vi "Process Menu Selection.vi"(8 "error in (no error)":errorcluster, 10 "Argument":string, 11 "Menu Ref":refnum<k9>) -> (0 "error out":errorcluster, 3 "State(s) to Enqueue":string)   [LabVIEW 2020, in "VI Properties Editor.lvlib"]
doc: "Processes a menu selection that occurred within the main window."
uses:
  VI Properties Editor.lvlib
  <vilib>/Utility/error.llb/Error Cluster From Error Code.vi
  <vilib>/ErrorRing/Error Ring.xnode
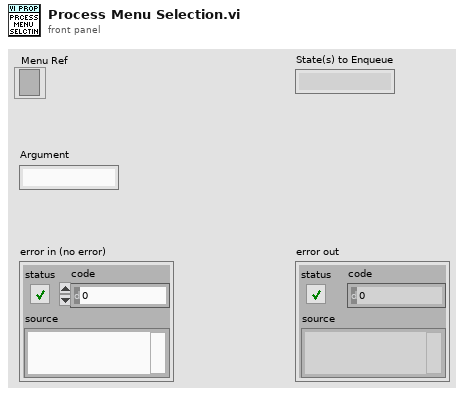
[diagram p1: front panel]
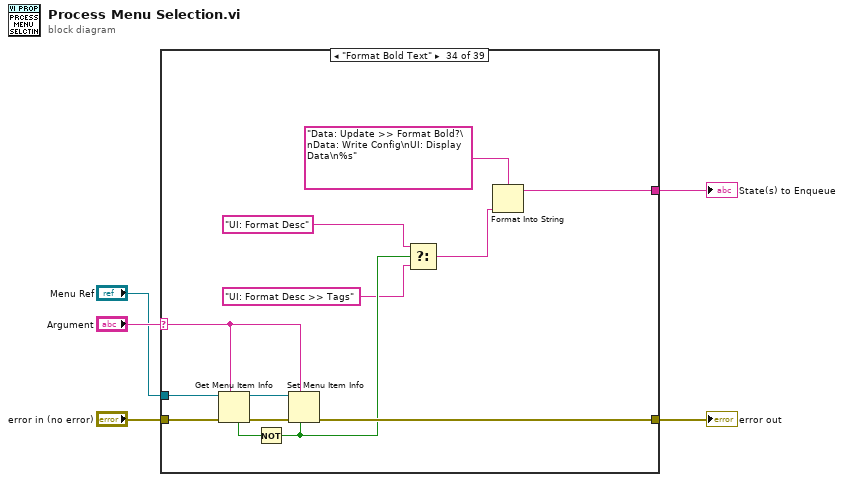
[diagram p0: block diagram]
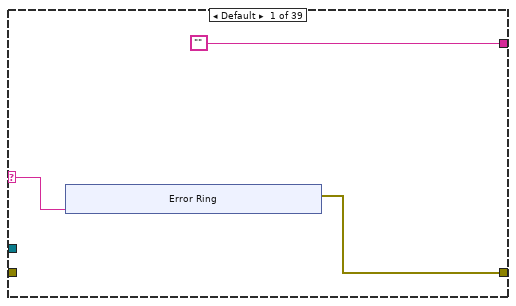
[diagram p2: hidden frame]
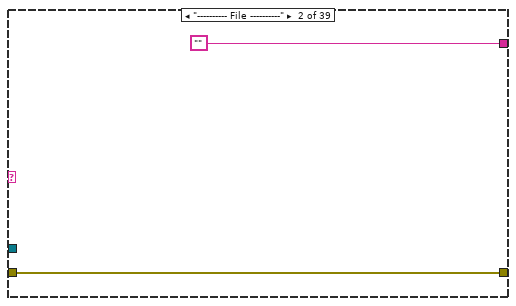
[diagram p3: hidden frame]
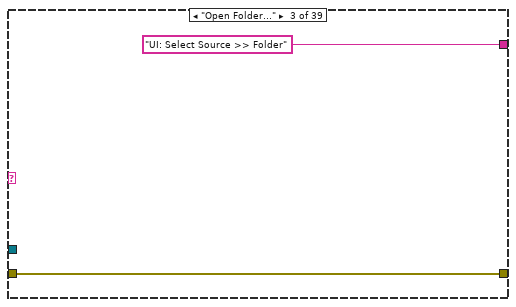
[diagram p4: hidden frame]
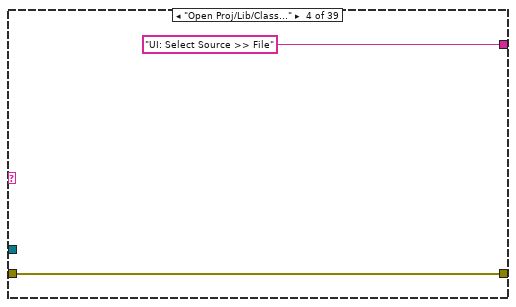
[diagram p5: hidden frame]
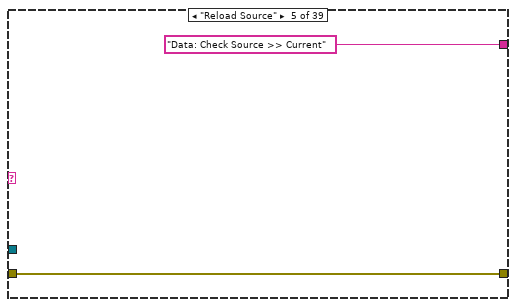
[diagram p6: hidden frame]
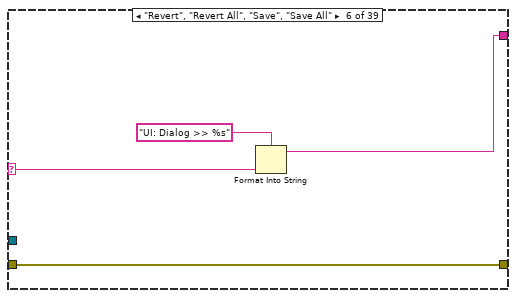
[diagram p7: hidden frame]
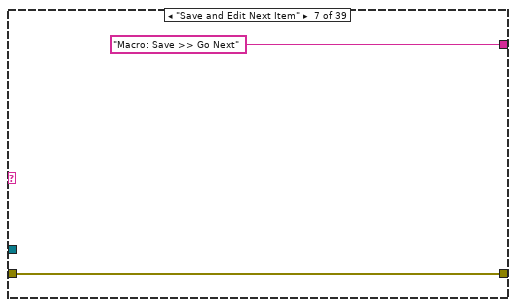
[diagram p8: hidden frame]
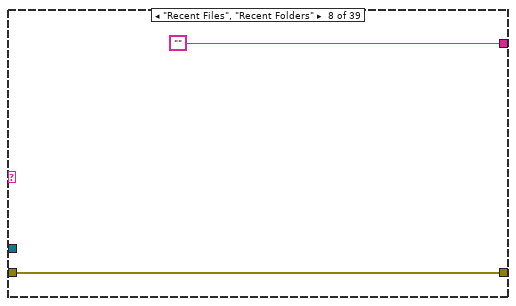
[diagram p9: hidden frame]
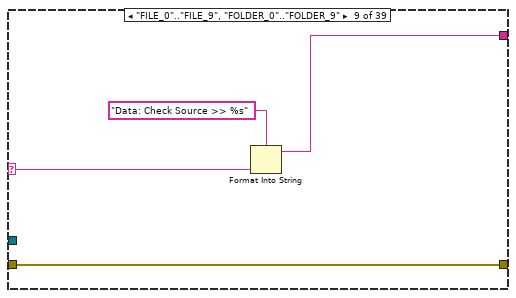
[diagram p10: hidden frame]
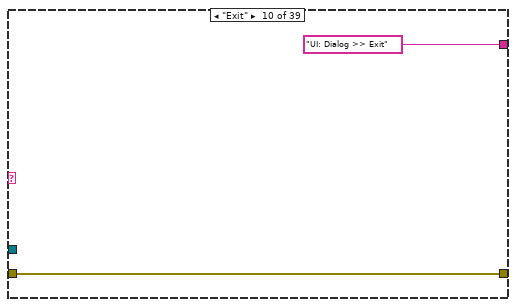
[diagram p11: hidden frame]
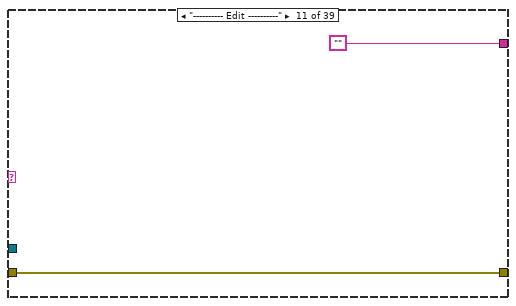
[diagram p12: hidden frame]
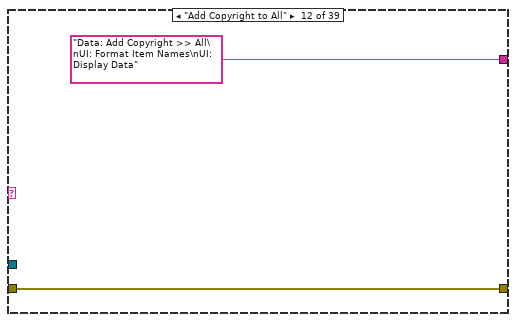
[diagram p13: hidden frame]
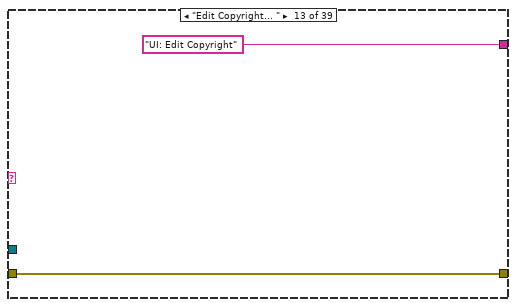
[diagram p14: hidden frame]
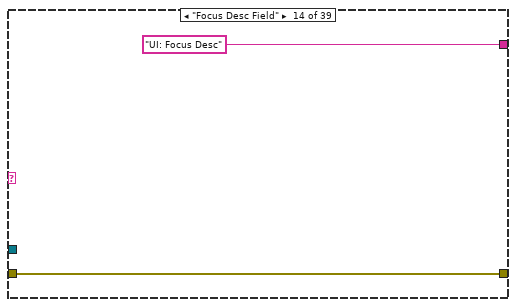
[diagram p15: hidden frame]
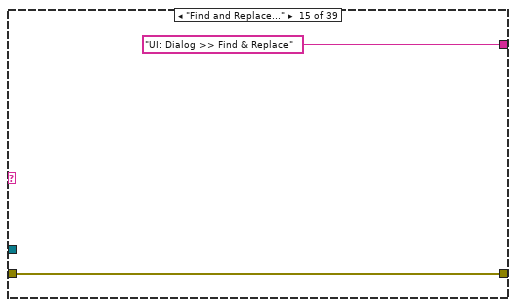
[diagram p16: hidden frame]
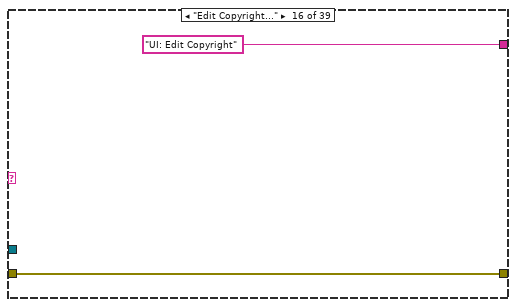
[diagram p17: hidden frame]
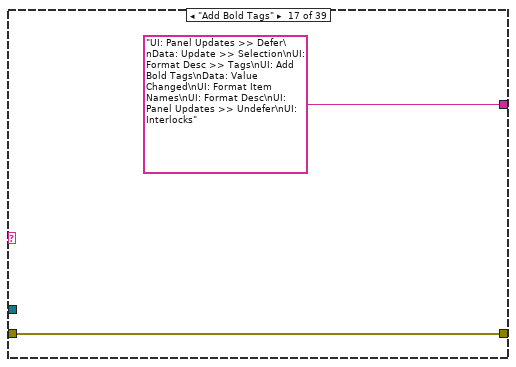
[diagram p18: hidden frame]
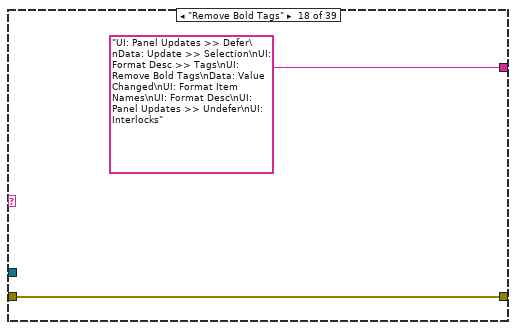
[diagram p19: hidden frame]
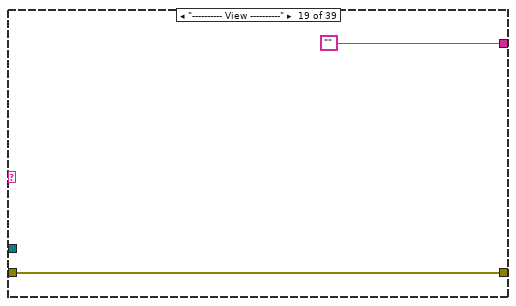
[diagram p20: hidden frame]
diagram:
  n1 = case shown="\"Format Bold Text\"" "Argument" {
    selector: "Argument" -> [w6 _ _ _ _ w25 _ _ w32 _ _ _ _ _ _ _ _ _ _ w61 w70 w79 _ w86 _ w107 w117 w121 w136 w145 w148 _ w165 w179 w188 w197 _ _ _]
    tunnel: ["" "" "UI: Select Source >> Folder" "UI: Select Source >> File" "Data: Check Source >> Current" w24 "Macro: Save >> Go Next" "" w33 "UI: Dialog >> Exit" "" "Data: Add Copyright >> All\nUI: Format Item Names\nUI: Display Data" "UI: Edit Copyright" "UI: Focus Desc" "UI: Dialog >> Find & Replace" "UI: Edit Copyright" "UI: Panel Updates >> Defer\nData: Update >> Selection\nUI: Format Desc >> Tags\nUI: Add Bold Tags\nData: Value Changed\nUI: Format Item Names\nUI: Format Desc\nUI: Panel Updates >> Undefer\nUI: Interlocks" "UI: Panel Updates >> Defer\nData: Update >> Selection\nUI: Format Desc >> Tags\nUI: Remove Bold Tags\nData: Value Changed\nUI: Format Item Names\nUI: Format Desc\nUI: Panel Updates >> Undefer\nUI: Interlocks" "" "Data: Update >> Filter\nData: Filter/Sort VIs\nData: Update >> Post-Filter VI\nUI: Format Item Names\nMacro: Load VI" "Data: Update >> Filter 2\nData: Filter/Sort VIs\nData: Update >> Post-Filter VI\nUI: Format Item Names\nMacro: Load VI" "Data: Update >> Clear Filter\nData: Filter/Sort VIs\nData: Update >> Post-Filter VI\nUI: Format Item Names\nMacro: Load VI" "UI: Dialog >> Custom Filter" "Data: Update >> Filter Config\nData: Write Config\nUI: Initialize Menu\nData: Filter/Sort VIs\nData: Update >> Post-Filter VI\nUI: Format Item Names\nMacro: Load VI" "" w109 "Data: Update >> Filter Data Source\nData: Filter/Sort VIs\nData: Update >> Post-Filter VI\nUI: Format Item Names\nMacro: Load VI" w120 "Data: Update >> Unsort\nData: Filter/Sort VIs\nData: Update >> Post-Filter VI\nUI: Format Item Names\nMacro: Load VI" "Data: Update >> Sort Order\nData: Filter/Sort VIs\nData: Update >> Post-Filter VI\nUI: Format Item Names\nMacro: Load VI" "Data: Update >> Flat View?\nData: Write Config\nData: Filter/Sort VIs\nData: Update >> Post-Filter VI\nUI: Format Item Names\nMacro: Load VI" "" "Data: Update >> Abbr Names?\nUI: Format Item Names\nData: Write Config" w170 "Data: Update >> ShowCPCtlsOnly?\nData: Write Config\nData: Update >> All Ctls\nUI: Display Data" "Data: Update >> ShowTLCtlsOnly?\nData: Write Config\nData: Update >> All Ctls\nUI: Display Data" "UI: Dialog >> Options" "" "UI: Dialog >> About"] -> w5
    tunnel: "Menu Ref" -> [_ _ _ _ _ _ _ _ _ _ _ _ _ _ _ _ _ _ _ w58 w67 w77 _ w92 _ w98 w118 w125 w137 w146 w149 _ w166 w180 w189 w198 _ _ _]
    tunnel: "error in (no error)" -> [_ w16 w18 w20 w22 w27 w28 w30 w35 w37 w39 w40 w42 w44 w46 w48 w50 w52 w55 w62 w71 w80 w83 w94 w96 w101 w112 w126 w135 w142 w151 w158 w160 w175 w184 w193 w199 w202 w203]
    tunnel: [w7 w16 w18 w20 w22 w27 w28 w30 w35 w37 w39 w40 w42 w44 w46 w48 w50 w52 w55 w60 w69 w74 w83 w89 w96 w100 w111 w129 w134 w141 w150 w158 w159 w174 w183 w192 w199 w202 w203] -> w4
    frame Default {
      n2 = xnode "Error Ring"("parameter 0"=w6) -> ("error out"=w7:errorcluster)
    }
    frame "---------- File ----------" {
    }
    frame "Open Folder..." {
    }
    frame "Open Proj/Lib/Class..." {
    }
    frame "Reload Source" {
    }
    frame "Revert", "Revert All", "Save", "Save All" {
      n3 = Format Into String(format string="UI: Dialog >> %s", w25) -> (resulting string=w24:string)  [unwired: 2 in, 1 out]
    }
    frame "Save and Edit Next Item" {
    }
    frame "Recent Files", "Recent Folders" {
    }
    frame "FILE_0".."FILE_9", "FOLDER_0".."FOLDER_9" {
      n4 = Format Into String(format string="Data: Check Source >> %s", w32) -> (resulting string=w33:string)  [unwired: 2 in, 1 out]
    }
    frame "Exit" {
    }
    frame "---------- Edit ----------" {
    }
    frame "Add Copyright to All" {
    }
    frame "Edit Copyright... " {
    }
    frame "Focus Desc Field" {
    }
    frame "Find and Replace..." {
    }
    frame "Edit Copyright..." {
    }
    frame "Add Bold Tags" {
    }
    frame "Remove Bold Tags" {
    }
    frame "---------- View ----------" {
    }
    frame "FILTER_NoDesc" {
      n5 = call "Uncheck Submenu Items.vi"("Item Tag"="Filter by", "error in (no error)"=w62, "Menu Ref"=w58) -> ("error out"=w59:errorcluster, "Menu Ref out"=w57:refnum<k9>)  [unwired: 7 in]
      n6 = Set Menu Item Info(6:TRUE ("checked"), 7:w61, 8:w59, 11:w57) -> (0:w60:errorcluster)  [unwired: 3 in, 1 out]
    }
    frame "FILTER_NoCtlCallouts" {
      n7 = call "Uncheck Submenu Items.vi"("Item Tag"="Filter by", "error in (no error)"=w71, "Menu Ref"=w67) -> ("error out"=w68:errorcluster, "Menu Ref out"=w66:refnum<k9>)  [unwired: 7 in]
      n8 = Set Menu Item Info(6:TRUE ("checked"), 7:w70, 8:w68, 11:w66) -> (0:w69:errorcluster)  [unwired: 3 in, 1 out]
    }
    frame "FILTER_Unfiltered" {
      n9 = call "Uncheck Submenu Items.vi"("Item Tag"="Filter by", "error in (no error)"=w80, "Menu Ref"=w77) -> ("error out"=w78:errorcluster, "Menu Ref out"=w76:refnum<k9>)  [unwired: 7 in]
      n10 = Set Menu Item Info(6:TRUE ("checked"), 7:w79, 8:w78, 11:w76) -> (0:w74:errorcluster)  [unwired: 3 in, 1 out]
    }
    frame "FILTER_Custom" {
    }
    frame "FILTER_Custom_Do" {
      n11 = call "Uncheck Submenu Items.vi"("Item Tag"="Filter by", "error in (no error)"=w94, "Menu Ref"=w92) -> ("error out"=w93:errorcluster, "Menu Ref out"=w91:refnum<k9>)  [unwired: 7 in]
      n12 = Search/Split String(string=w86, search string/char (-)="_Do") -> (substring before match=w85:string)  [unwired: 1 in, 2 out]
      n13 = Set Menu Item Info(6:TRUE ("checked"), 7:w85, 8:w93, 11:w91) -> (0:w89:errorcluster)  [unwired: 3 in, 1 out]
    }
    frame "Recent Filters" {
    }
    frame "FILTER_0".."FILTER_9" {
      n14 = Search/Split String(string=w107, search string/char (-)="_") -> (substring before match=w108:string)  [unwired: 1 in, 2 out]
      n15 = call "Uncheck Submenu Items.vi"("Item Tag"="Filter by", "error in (no error)"=w101, "Menu Ref"=w98) -> ("error out"=w105:errorcluster, "Menu Ref out"=w104:refnum<k9>)  [unwired: 7 in]
      n16 = Format Into String(format string="Data: Update >> %s\nData: Update >> %s Config\nData: Write Config\nUI: Initialize Menu\nData: Filter/Sort VIs\nData: Update >> Post-Filter VI\nUI: Format Item Names\nMacro: Load VI", w107, w108) -> (resulting string=w109:string)  [unwired: 2 in, 1 out]
      n17 = Set Menu Item Info(6:TRUE ("checked"), 7:"FILTER_Custom" ("item tag"), 8:w105, 11:w104) -> (0:w100:errorcluster)  [unwired: 3 in, 1 out]
    }
    frame "FILTER_DataSource" {
      n18 = Get Menu Item Info(7:w117, 8:w112, 11:w118) -> (0:w116:errorcluster, 3:w115:refnum<k9>, 4:w114:bool)  [unwired: 4 out]
      n19 = Not(x=w114) -> (.not. x?=w113:bool)
      n20 = Set Menu Item Info(6:w113, 7:w117, 8:w116, 11:w115) -> (0:w111:errorcluster)  [unwired: 3 in, 1 out]
    }
    frame "SORT_0".."SORT_99" {
      n21 = call "Uncheck Submenu Items.vi"("Item Tag"="Sort by" ("item tag"), "error in (no error)"=w126, "Menu Ref"=w125) -> ("error out"=w123:errorcluster, "Menu Ref out"=w124:refnum<k9>)  [unwired: 7 in]
      n22 = Set Menu Item Info(6:TRUE ("checked"), 7:w121, 8:w123, 11:w124) -> (0:w129:errorcluster)  [unwired: 3 in, 1 out]
      n23 = Format Into String(format string="Data: Update >> %s\nData: Filter/Sort VIs\nData: Update >> Post-Filter VI\nUI: Format Item Names\nMacro: Load VI", w121) -> (resulting string=w120:string)  [unwired: 2 in, 1 out]
    }
    frame "SORT_Unsorted" {
      n24 = call "Uncheck Submenu Items.vi"("Item Tag"="Sort by" ("item tag"), "error in (no error)"=w135, "Menu Ref"=w137) -> ("error out"=w130:errorcluster, "Menu Ref out"=w131:refnum<k9>)  [unwired: 7 in]
      n25 = Set Menu Item Info(6:TRUE ("checked"), 7:w136, 8:w130, 11:w131) -> (0:w134:errorcluster)  [unwired: 3 in, 1 out]
    }
    frame "SORT_Order" {
      n26 = Get Menu Item Info(7:w145, 8:w142, 11:w146) -> (0:w144:errorcluster, 3:w143:refnum<k9>, 4:w140:bool)  [unwired: 4 out]
      n27 = Not(x=w140) -> (.not. x?=w139:bool)
      n28 = Set Menu Item Info(6:w139, 7:w145, 8:w144, 11:w143) -> (0:w141:errorcluster)  [unwired: 3 in, 1 out]
    }
    frame "FLAT" {
      n29 = Get Menu Item Info(7:w148, 8:w151, 11:w149) -> (0:w155:errorcluster, 3:w154:refnum<k9>, 4:w153:bool)  [unwired: 4 out]
      n30 = Not(x=w153) -> (.not. x?=w152:bool)
      n31 = Set Menu Item Info(6:w152, 7:w148, 8:w155, 11:w154) -> (0:w150:errorcluster)  [unwired: 3 in, 1 out]
    }
    frame "---------- Options ----------" {
    }
    frame "Abbr if Class in Lib" {
      n32 = Get Menu Item Info(7:w165, 8:w160, 11:w166) -> (0:w164:errorcluster, 3:w163:refnum<k9>, 4:w162:bool)  [unwired: 4 out]
      n33 = Not(x=w162) -> (.not. x?=w161:bool)
      n34 = Set Menu Item Info(6:w161, 7:w165, 8:w164, 11:w163) -> (0:w159:errorcluster)  [unwired: 3 in, 1 out]
    }
    frame "Format Bold Text" {
      n35 = Get Menu Item Info(7:w179, 8:w175, 11:w180) -> (0:w178:errorcluster, 3:w177:refnum<k9>, 4:w176:bool)  [unwired: 4 out]
      n36 = Not(x=w176) -> (.not. x?=w173:bool)
      n37 = Set Menu Item Info(6:w173, 7:w179, 8:w178, 11:w177) -> (0:w174:errorcluster)  [unwired: 3 in, 1 out]
      n38 = Select(t="UI: Format Desc", s=w173, f="UI: Format Desc >> Tags") -> (s? t:f=w168:string)
      n39 = Format Into String(format string="Data: Update >> Format Bold?\nData: Write Config\nUI: Display Data\n%s", w168) -> (resulting string=w170:string)  [unwired: 2 in, 1 out]
    }
    frame "Only Show ConPane Ctls" {
      n40 = Get Menu Item Info(7:w188, 8:w184, 11:w189) -> (0:w187:errorcluster, 3:w186:refnum<k9>, 4:w185:bool)  [unwired: 4 out]
      n41 = Not(x=w185) -> (.not. x?=w182:bool)
      n42 = Set Menu Item Info(6:w182, 7:w188, 8:w187, 11:w186) -> (0:w183:errorcluster)  [unwired: 3 in, 1 out]
    }
    frame "Only Show Top-Level Ctls" {
      n43 = Get Menu Item Info(7:w197, 8:w193, 11:w198) -> (0:w196:errorcluster, 3:w195:refnum<k9>, 4:w194:bool)  [unwired: 4 out]
      n44 = Not(x=w194) -> (.not. x?=w191:bool)
      n45 = Set Menu Item Info(6:w191, 7:w197, 8:w196, 11:w195) -> (0:w192:errorcluster)  [unwired: 3 in, 1 out]
    }
    frame "All Options..." {
    }
    frame "---------- Help ----------" {
    }
    frame "About..." {
    }
  }
  "error out" <- w4
  "State(s) to Enqueue" <- w5
